vi "Dateiname mit Zeitstempel.vi"(8 "genaue Zeit":bool, 10 "Extension in":string, 11 "File Name in":string) -> (3 "File Name":string)   [LabVIEW 2020, in "allgemeine Sub-VIs.lvlib"]
doc: "Hängt dem angegebenen Dateinamen einen Zeitstempel an, bei dem die Sonderzeichen Verzeichnis kompatibel ersetzt wurden + extension.\nriw 8.6.2018"
uses:
  allgemeine Sub-VIs.lvlib
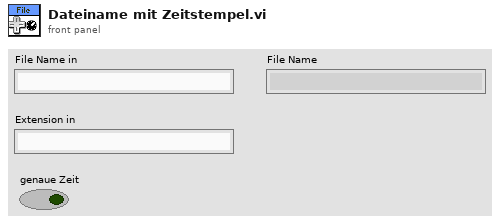
[diagram p1: front panel]
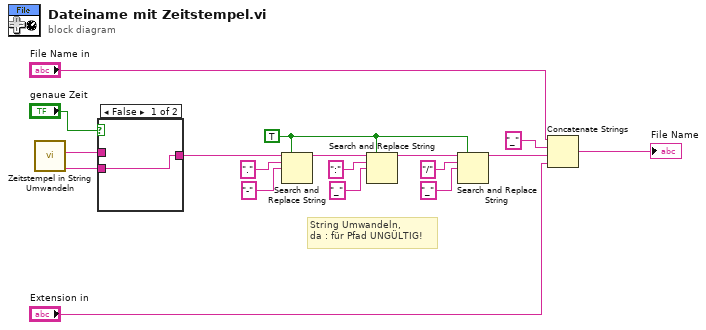
[diagram p0: block diagram]
diagram:
  w9 = TRUE ("Alle ersetzen? (F)")
  # "String Umwandeln, \nda : für Pfad UNGÜLTIG!"
  n1 = call "Zeitstempel in String Umwandeln.vi"() -> ("Zeitstempel"=w2:string, "Zeitstempel mit Kommastellen"=w3:string)  [unwired: 10 in]
  n2 = case shown="False" "genaue Zeit" {
    tunnel: w3 -> [_ w20]
    tunnel: w2 -> [w19 _]
    tunnel: [w19 w20] -> w1
    frame False {
    }
    frame True {
    }
  }
  n3 = Search and Replace String(replace all?=w9, input string=w1, search string="." ("Such-String"), replace string="-" ("String ersetzen(\"\")")) -> (result string=w16:string)  [unwired: 4 in, 3 out]
  n4 = Search and Replace String(replace all?=w9, input string=w16, search string=":" ("Such-String"), replace string="_" ("String ersetzen(\"\")")) -> (result string=w10:string)  [unwired: 4 in, 3 out]
  n5 = Search and Replace String(replace all?=w9, input string=w10, search string="/" ("Such-String"), replace string="_" ("String ersetzen(\"\")")) -> (result string=w8:string)  [unwired: 4 in, 3 out]
  n6 = Concatenate Strings("File Name in", "_", w8, "Extension in") -> (→"File Name":string)
